vi "Tricomi Function.vi"(3 "b":dbl format="%.2f", 4 "a":dbl format="%.2f", 5 "x":dbl format="%.2f") -> (2 "U(x, a, b)":dbl format="%.2f")   [LabVIEW 2010, in "NI_Gmath.lvlib"]
doc: "Computes the Tricomi, or associated confluent hypergeometric, function."
uses:
  NI_Gmath.lvlib
  lvanlys.dll
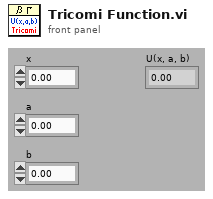
[diagram p1: front panel]
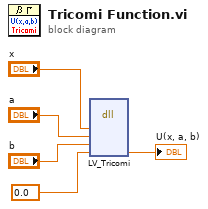
[diagram p0: block diagram]
diagram:
  n1 = dll-call lib="C:/Program Files/National Instruments/LabVIEW 2010/resource/lvanlys.*" fn="LV_Tricomi"("x"="x", "a"="a", "b"="b", "Tricomi(x, a, b)"=0.0 ("Kummer")) -> ("Tricomi(x, a, b)"=→"U(x, a, b)":dbl)  [unwired: 7 in, 2 out]
